vi "Widefield_Main.vi"() -> ()   [LabVIEW 2012]
doc: "Main window for the new intrinsic imaging setup.\nAntoniu Fantana, 2003\n\nThis is a sequence (init, main loop, save logbook, exit program), where the most time\nwill be spent inside the main loop."
uses:
  Widefield_globals.vi
panel:
  in  "Start":bool caption="OK Button"
  in  "Focus Camera":bool
  in  "Settings":bool
  in  "Load Experiment":bool
  in  "stop":bool
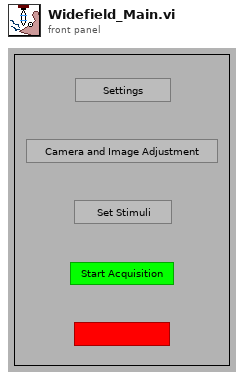
[diagram p1: front panel]
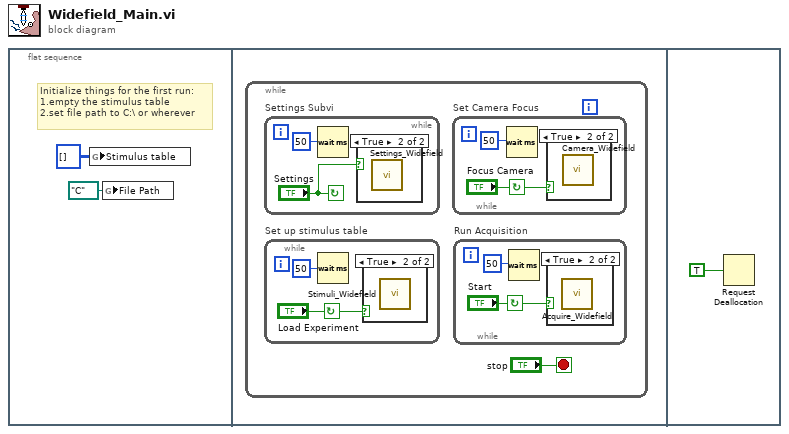
[diagram p0: block diagram]
diagram:
  n1 = flat-sequence {
    frame #0 {
      # "Initialize things for the first run:\n1.empty the stimulus table\n2.set file path to C:\\ or wherever"
      n2 = global write "Widefield_globals.vi" "Stimulus table"(i32[][] []) -> ()
      n3 = global write "Widefield_globals.vi" "File Path"(path "C:/" ("File Path")) -> ()
    }
    frame #1 {
      n4 = while {
        stop <- "stop" stop-if-true
        n5 = while "Settings Subvi" {
          stop <- "Settings" continue-if-true
          n6 = Wait (ms)(milliseconds to wait=50) -> ()  [unwired: 1 out]
          n7 = case shown="True" "Settings" {
            frame False {
            }
            frame True {
              n8 = call "Settings_Widefield.vi"() -> ()  [unwired: 1 in]
            }
          }
        }
        n9 = while "Set up stimulus table" {
          stop <- "Load Experiment" continue-if-true
          n10 = Wait (ms)(milliseconds to wait=50) -> ()  [unwired: 1 out]
          n11 = case shown="True" "Load Experiment" {
            frame False {
            }
            frame True {
              n12 = call "Stimuli_Widefield.vi"() -> ()  [unwired: 1 in]
            }
          }
        }
        n13 = while "Set Camera Focus" {
          stop <- "Focus Camera" continue-if-true
          n14 = Wait (ms)(milliseconds to wait=50) -> ()  [unwired: 1 out]
          n15 = case shown="True" "Focus Camera" {
            frame False {
            }
            frame True {
              n16 = call "Camera_Widefield.vi"() -> ()  [unwired: 12 in]
            }
          }
        }
        n17 = while "Run Acquisition" {
          stop <- "Start" continue-if-true
          n18 = Wait (ms)(milliseconds to wait=50) -> ()  [unwired: 1 out]
          n19 = case shown="True" "Start" {
            frame False {
            }
            frame True {
              n20 = call "Acquire_Widefield.vi"() -> ()  [unwired: 1 in]
            }
          }
        }
      }
    }
    frame #2 {
      n21 = Request Deallocation(TRUE ("flag")) -> ()
    }
  }
